vi "Encode.vi"(8 "Error in":errorcluster, 11 "Decoded message":u8[](array[numeric]) format="%02x") -> (0 "Error out":errorcluster, 3 "Encoded message":u8[](array[numeric]) format="%02x")   [LabVIEW 2020, in "COBS.lvlib"]
uses:
  COBS.lvlib
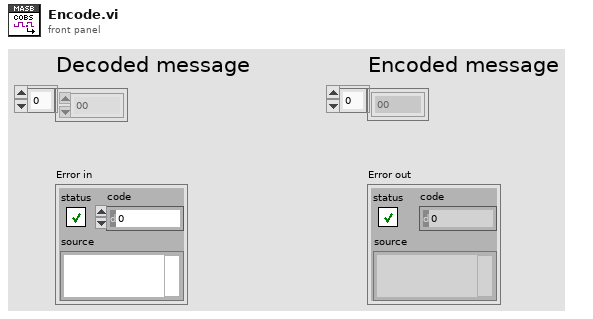
[diagram p1: front panel]
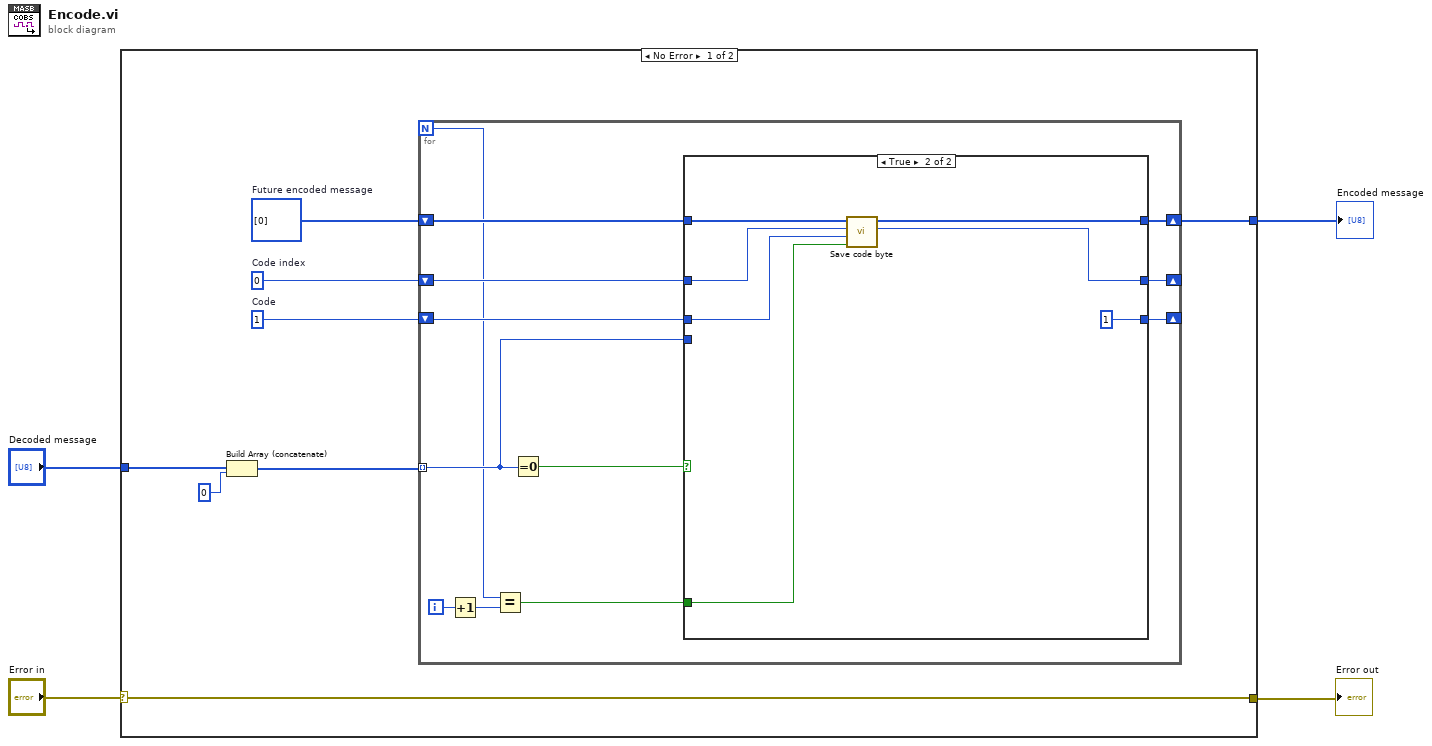
[diagram p0: block diagram]
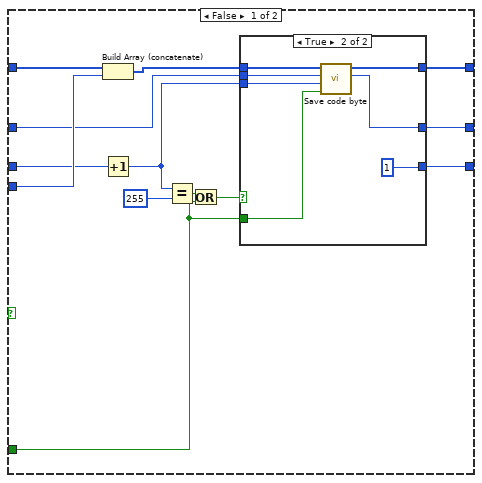
[diagram p2: hidden frame]
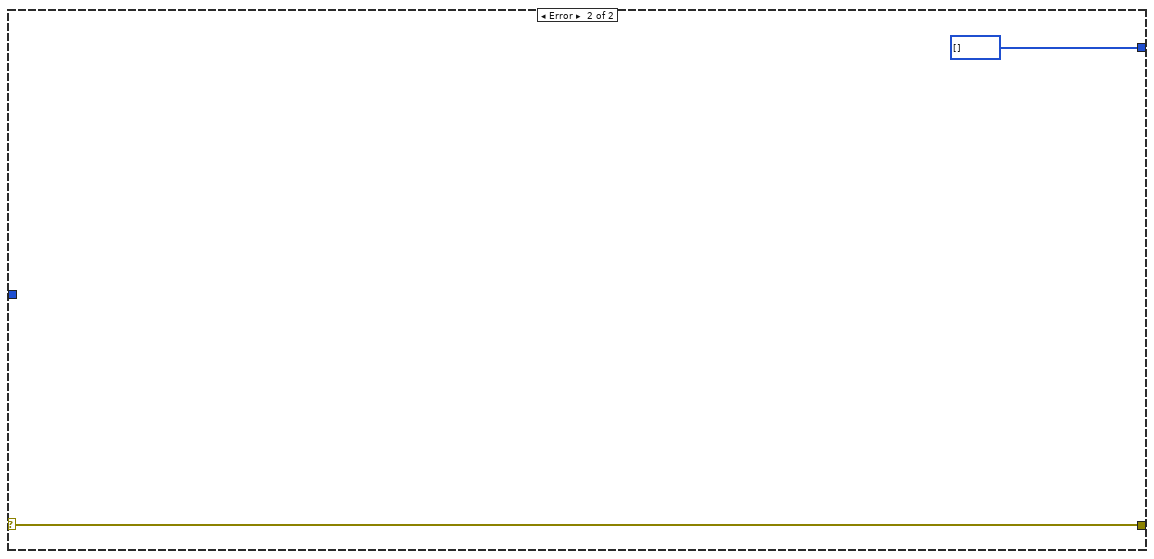
[diagram p4: hidden frame]
diagram:
  n1 = case shown="No Error" "Error in" {
    selector: "Error in" -> [w12 w56]
    tunnel: [w12 w56] -> w3
    tunnel: "Decoded message" -> [w7 _]
    tunnel: [w8 u8[] []] -> w1
    frame No Error {
      w9 = 0  # Code index
      w10 = u8[] [0]  # Future encoded message
      w11 = u8 1  # Code
      n2 = Build Array (concatenate)(w7, u8 0) -> (w5:u8[])
      n3 = for {
        N -> [w14]
        tunnel: w5 -> [w18] mode=indexing
        shift-right: [w23] -> _
        shift-left: w11 -> [w22]
        shift-right: [w19] -> w8
        shift-left: w10 -> [w21]
        shift-right: [w17] -> _
        shift-left: w9 -> [w20]
        i -> [w16]
        n4 = Increment(x=w16) -> (x+1=w15:i32)
        n5 = Equal?(x=w14, y=w15) -> (x = y?=w13:bool)
        n6 = Equal To 0?(x=w18) -> (x = 0?=w24:bool)
        n7 = case shown="True" w24 {
          tunnel: [w29 u8 1 ("Code")] -> w23
          tunnel: w22 -> [w35 w52]
          tunnel: w21 -> [w37 w54]
          tunnel: w20 -> [w32 w53]
          tunnel: [w31 w49] -> w19
          tunnel: w18 -> [w36 _]
          tunnel: [w30 w50] -> w17
          tunnel: w13 -> [w25 w48]
          frame False {
            n8 = Build Array (concatenate)(w37, w36) -> (w33:u8[])
            n9 = Increment(x=w35) -> (x+1=w28:u8)
            n10 = Equal?(x=w28, y=u8 255) -> (x = y?=w27:bool)
            n11 = Or(x=w27, y=w25) -> (x .or. y?=w26:bool)
            n12 = case shown="True" w26 {
              tunnel: w33 -> [w39 w46]
              tunnel: w32 -> [w38 w43]
              tunnel: [w39 w45] -> w31
              tunnel: [w38 w44] -> w30
              tunnel: [w40 u8 1] -> w29
              tunnel: w28 -> [w40 w42]
              tunnel: w25 -> [_ w41]
              frame False {
              }
              frame True {
                n13 = call "Save code byte.vi"("Last buffer element?"=w41, "Code"=w42, "Code index in"=w43, "Buffer in"=w46) -> ("Code index out"=w44:i32, "Buffer out"=w45:u8[])  [unwired: 6 in]
              }
            }
          }
          frame True {
            n14 = call "Save code byte.vi"("Last buffer element?"=w48, "Code"=w52, "Code index in"=w53, "Buffer in"=w54) -> ("Code index out"=w50:i32, "Buffer out"=w49:u8[])  [unwired: 6 in]
          }
        }
      }
    }
    frame Error {
    }
  }
  "Error out" <- w3
  "Encoded message" <- w1
